vi "Get User Input.vi"(10 "OK Button Text":string, 11 "Sequence Context In":refnum<k7>) -> (1 "Continue Testing?":bool, 2 "UUT Data":T2)   [LabVIEW 2010]
uses:
  TouchScreen UI Elements/_TypeDefs/OK Button_TouchScreen.ctl
  Data to Validate.ctl
  <vilib>/addons/TestStand/_TSUtility.llb/TestStand - Get Property Value (String).vi
panel:
  in  "Work Order Number":string
  in  "QiG Serial Number":string
  in  "UUT Part Number":string
  in  "Cancel Button":T1
  in  "Continue Button":T1
  in  "UUT MICS ID":u32 format="%06x"
  in  "UUT Serial Number":string
  in  "UUT Lot Number":string
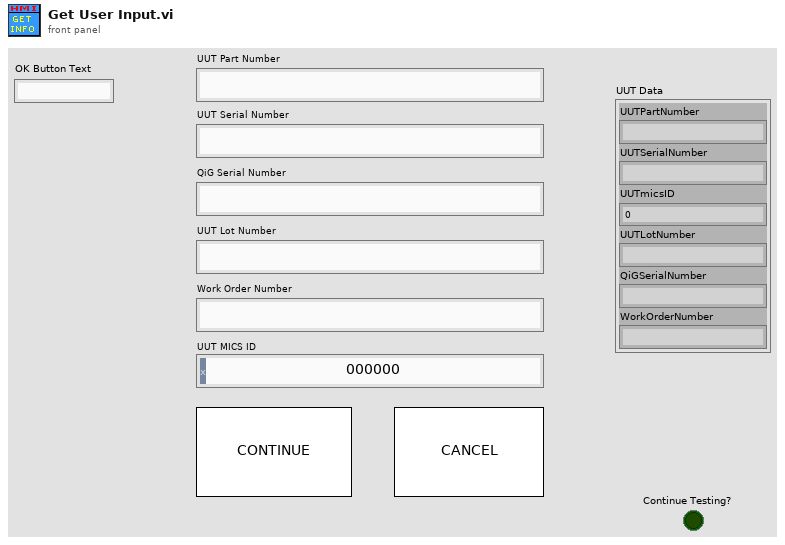
[diagram p1: front panel]
types:
  T1 = typedef "OK Button_TouchScreen.ctl" = bool
  T2 = cluster{"UUTmicsID":u32, "UUTLotNumber":string, "UUTSerialNumber":string, "UUTPartNumber":string, "QiGSerialNumber":string, "WorkOrderNumber":string}
  T3 = enum32{"Invalid", "Standard", "Closed", "Hidden", "Minimized", "Maximized"}
  T4 = typedef "Data to Validate.ctl" = enum16{"UUT_Part_Number", "UUT_Serial_Number", "QiG_Serial_Number", "UUT_Model_Number", "UUT_Lot_Number", "Work_Order_Number", "UUT_MICS_ID"}
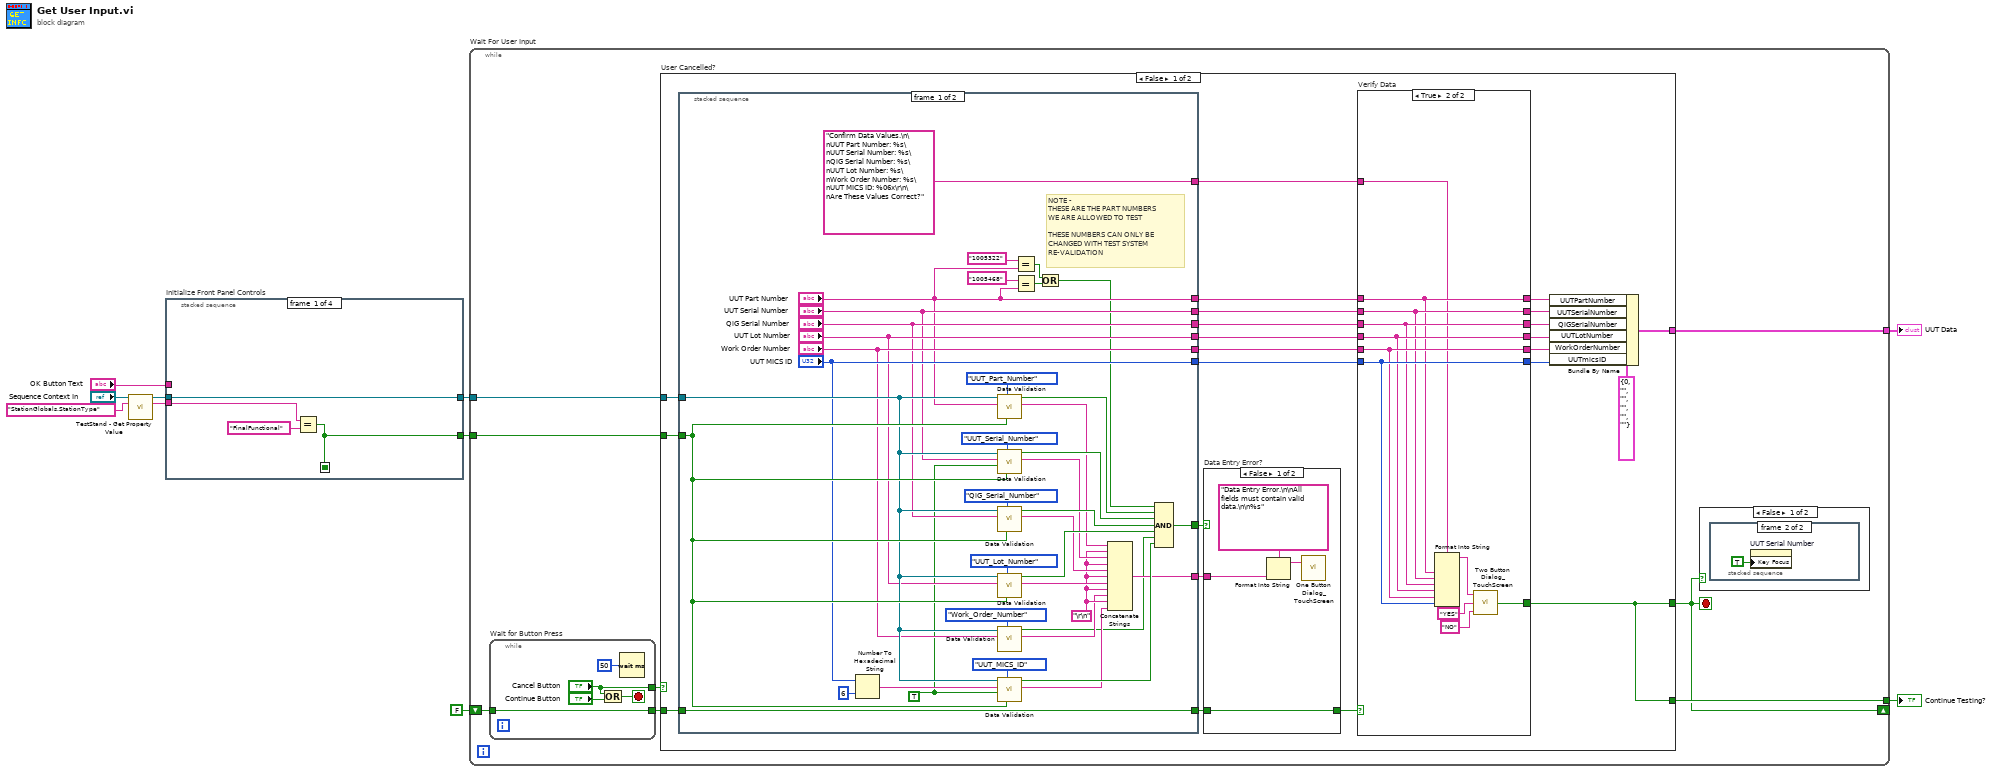
[diagram p0: block diagram]
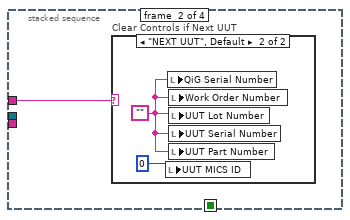
[diagram p2: hidden frame]
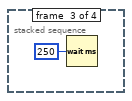
[diagram p4: hidden frame]
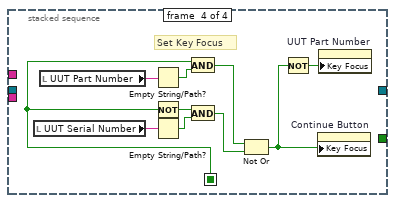
[diagram p5: hidden frame]
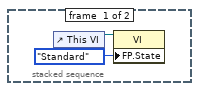
[diagram p6: hidden frame]
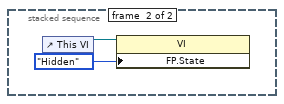
[diagram p8: hidden frame]
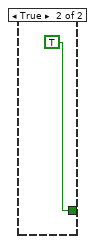
[diagram p10: hidden frame]
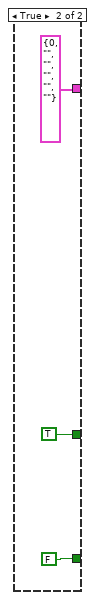
[diagram p11: hidden frame]
diagram:
  n1 = call-poly <vilib>:"TestStand - Get Property Value.vi"("Sequence Context In"="Sequence Context In", "Lookup String"="StationGlobals.StationType") -> ("Sequence Context Out"=w4:refnum<k7>, "Value"=w3:string)  [unwired: 11 in, 1 out]
  n2 = stacked-sequence "Initialize Front Panel Controls" {
    seq-local: [w11 _ _ _] -> [_ _ _ w24]
    tunnel: "OK Button Text" -> [_ w15 _ _]
    tunnel: w4 -> [w14 _ _ _]
    tunnel: w3 -> [w13 _ _ _]
    tunnel: [w14 _ _ _] -> w2
    tunnel: [w11 _ _ _] -> w1
    frame #0 {
      n3 = Equal?(x=w13, y="FinalFunctional") -> (x = y?=w11:bool)
    }
    frame #1 {
      n4 = case "Clear Controls if Next UUT" shown="\"NEXT UUT\", Default" w15 {
        frame "RETEST" {
        }
        frame "NEXT UUT", Default {
          w16 = "" ("Device LOT Number")
          n5 = local write "UUT MICS ID"(u32 0 ("Device MICS ID")) -> ()
          n6 = local write "QiG Serial Number"(w16) -> ()
          n7 = local write "Work Order Number"(w16) -> ()
          n8 = local write "UUT Lot Number"(w16) -> ()
          n9 = local write "UUT Serial Number"(w16) -> ()
          n10 = local write "UUT Part Number"(w16) -> ()
        }
      }
    }
    frame #2 {
      n11 = Wait (ms)(milliseconds to wait=u32 250) -> ()  [unwired: 1 out]
    }
    frame #3 {
      # "Set Key Focus"
      n12 = local read "UUT Serial Number"() -> (w26:string)
      n13 = local read "UUT Part Number"() -> (w27:string)
      n14 = Empty String/Path?(string/path=w27) -> (empty?=w28:bool)
      n15 = Not(x=w24) -> (.not. x?=w23:bool)
      n16 = Empty String/Path?(string/path=w26) -> (empty?=w25:bool)
      n17 = And(x=w24, y=w28) -> (x .and. y?=w21:bool)
      n18 = And(x=w23, y=w25) -> (x .and. y?=w22:bool)
      n19 = Not Or(1:w22, 2:w21) -> (0:w19:bool)
      n20 = Not(x=w19) -> (.not. x?=w20:bool)
      n21 = property on="Continue Button" class="Bool"("Key Focus"=w19) -> ()  [unwired: 2 in, 2 out]
      n22 = property on="UUT Part Number" class="Str"("Key Focus"=w20) -> ()  [unwired: 2 in, 2 out]
    }
  }
  n23 = while "Wait For User Input" {
    shift-right: [w31] -> _
    shift-left: FALSE -> [w36]
    tunnel: [w34] -> w7
    tunnel: [w32] -> w9
    tunnel: w2 -> [w30]
    tunnel: w1 -> [w29]
    stop <- w31 stop-if-true
    n24 = while "Wait for Button Press" {
      tunnel: w36 -> [w134]
      tunnel: [w134] -> w35
      tunnel: ["Cancel Button"] -> w33
      stop <- w131 stop-if-true
      n25 = Or(x="Cancel Button", y="Continue Button") -> (x .or. y?=w131:T1)
      n26 = Wait (ms)(milliseconds to wait=u32 50) -> ()  [unwired: 1 out]
    }
    n27 = case "User Cancelled?" shown="False" w33 {
      tunnel: w35 -> [w61 _]
      tunnel: [w51 TRUE ("T button?")] -> w31
      tunnel: [w56 T2 {"UUTmicsID"=0, "UUTLotNumber"="", "UUTSerialNumber"="", "UUTPartNumber"="", "QiGSerialNumber"="", "WorkOrderNumber"=""} ("UUT Data")] -> w34
      tunnel: [w51 FALSE] -> w32
      tunnel: w30 -> [w49 _]
      tunnel: w29 -> [w46 _]
      frame False {
        n28 = stacked-sequence {
          tunnel: [w100 _] -> w62
          tunnel: ["UUT Serial Number" _] -> w57
          tunnel: ["UUT Lot Number" _] -> w58
          tunnel: ["UUT MICS ID" _] -> w54
          tunnel: w61 -> [w99 _]
          tunnel: [w99 _] -> w60
          tunnel: [w87 _] -> w50
          tunnel: w49 -> [w75 _]
          tunnel: ["UUT Part Number" _] -> w48
          tunnel: w46 -> [w81 _]
          tunnel: ["Confirm Data Values.\n\nUUT Part Number: %s\nUUT Serial Number: %s\nQiG Serial Number: %s\nUUT Lot Number: %s\nWork Order Number: %s\nUUT MICS ID: %06x\r\n\nAre These Values Correct?" ("format string") _] -> w45
          tunnel: ["QiG Serial Number" _] -> w44
          tunnel: ["Work Order Number" _] -> w43
          frame #0 {
            w78 = "\r\n"
            w63 = TRUE
            # "NOTE -\nTHESE ARE THE PART NUMBERS\nWE ARE ALLOWED TO TEST\n\nTHESE NUMBERS CAN ONLY BE\nCHANGED WITH TEST SYSTEM\nRE-VALIDATION"
            n29 = Number To Hexadecimal String(1:i16 6 ("width (-)"), 2:"UUT MICS ID") -> (0:w93:string)
            n30 = call "Data Validation.vi"("Final Functional Test Station?"=w81, "Input Data Descriptor"=Data_to_Validate."UUT_Part_Number", "Input to Validate"="UUT Part Number", "Sequence Context In"=w75) -> ("Message"=w85:string, "String Valid?"=w84:bool)  [unwired: 5 in, 1 out]
            n31 = call "Data Validation.vi"("Final Functional Test Station?"=w81, "Input Data Descriptor"=Data_to_Validate."UUT_Serial_Number", "Is HEX String?"=w63, "Input to Validate"="UUT Serial Number", "Sequence Context In"=w75) -> ("Message"=w90:string, "String Valid?"=w97:bool)  [unwired: 4 in, 1 out]
            n32 = call "Data Validation.vi"("Final Functional Test Station?"=w81, "Input Data Descriptor"=Data_to_Validate."QiG_Serial_Number", "Input to Validate"="QiG Serial Number", "Sequence Context In"=w75) -> ("Message"=w79:string, "String Valid?"=w101:bool)  [unwired: 5 in, 1 out]
            n33 = call "Data Validation.vi"("Final Functional Test Station?"=w81, "Input Data Descriptor"=Data_to_Validate."UUT_Lot_Number", "Input to Validate"="UUT Lot Number", "Sequence Context In"=w75) -> ("Message"=w89:string, "String Valid?"=w95:bool)  [unwired: 5 in, 1 out]
            n34 = call "Data Validation.vi"("Input Data Descriptor"=Data_to_Validate."Work_Order_Number", "Input to Validate"="Work Order Number", "Sequence Context In"=w75) -> ("Message"=w77:string, "String Valid?"=w76:bool)  [unwired: 6 in, 1 out]
            n35 = call "Data Validation.vi"("Final Functional Test Station?"=w81, "Input Data Descriptor"=Data_to_Validate."UUT_MICS_ID", "Is HEX String?"=w63, "Input to Validate"=w93, "Sequence Context In"=w75) -> ("Message"=w88:string, "String Valid?"=w91:bool)  [unwired: 4 in, 1 out]
            n36 = Equal?(x="1005322" ("Message"), y="UUT Part Number") -> (x = y?=w65:bool)
            n37 = Equal?(x="1005468" ("Message"), y="UUT Part Number") -> (x = y?=w66:bool)
            n38 = Or(x=w65, y=w66) -> (x .or. y?=w64:bool)
            n39 = Concatenate Strings(w85, w78, w90, w78, w79, w78, w89, w78, w77, w78, w88) -> (w87:string)
            n40 = Compound Arithmetic op=AND(w64, w84, w97, w101, w95, w76, w91) -> (w100:bool)
          }
          frame #1 {
            n41 = control-ref of="This VI"() -> (w103:refnum<vi>)
            n42 = property class="VI"(reference=w103, "FP.State"=T3."Hidden" ("Front Panel Window:State")) -> ()  [unwired: 1 in, 2 out]
          }
        }
        n43 = case "Data Entry Error?" shown="False" w62 {
          tunnel: w60 -> [w125 _]
          tunnel: [w125 TRUE] -> w59
          tunnel: w50 -> [w122 _]
          frame False {
            n44 = Format Into String(format string="Data Entry Error.\n\nAll fields must contain valid data.\n\n%s" ("message"), w122) -> (resulting string=w123:string)  [unwired: 2 in, 1 out]
            n45 = call "One Button Dialog_TouchScreen.vi"("Message"=w123) -> ()  [unwired: 1 in, 1 out]
          }
          frame True {
          }
        }
        n46 = case "Verify Data" shown="True" w59 {
          selector: w59 -> [w107 _]
          tunnel: w54 -> [w110 w117]
          tunnel: w58 -> [w109 w115]
          tunnel: w57 -> [w108 w113]
          tunnel: [w107 w118] -> w51
          tunnel: [w110 w117] -> w53
          tunnel: [w109 w115] -> w55
          tunnel: [w108 w113] -> w52
          tunnel: w48 -> [w106 w112]
          tunnel: [w106 w112] -> w47
          tunnel: w45 -> [_ w111]
          tunnel: w44 -> [w105 w114]
          tunnel: w43 -> [w104 w116]
          tunnel: [w105 w114] -> w40
          tunnel: [w104 w116] -> w41
          frame False {
          }
          frame True {
            n47 = Format Into String(format string=w111, w112, w113, w114, w115, w116, w117) -> (resulting string=w121:string)  [unwired: 2 in, 1 out]
            n48 = call "Two Button Dialog_TouchScreen.vi"("F button name (\"Cancel\")"="NO" ("F button name (\"Cancel\")"), "T button name (\"OK\")"="YES" ("T button name (\"OK\")"), "Message"=w121) -> ("T Button?"=w118:T1)
          }
        }
        n49 = Bundle By Name(cluster=T2 {"UUTmicsID"=0, "UUTLotNumber"="", "UUTSerialNumber"="", "UUTPartNumber"="", "QiGSerialNumber"="", "WorkOrderNumber"=""} ("UUT Data"), "UUTPartNumber"=w47, "UUTSerialNumber"=w52, "QiGSerialNumber"=w40, "UUTLotNumber"=w55, "WorkOrderNumber"=w41, "UUTmicsID"=w53) -> (w56:T2)
      }
      frame True {
      }
    }
    n50 = case shown="False" w31 {
      frame False {
        n51 = stacked-sequence {
          frame #0 {
            n52 = control-ref of="This VI"() -> (w38:refnum<vi>)
            n53 = property class="VI"(reference=w38, "FP.State"=T3."Standard" ("Front Panel Window:State")) -> ()  [unwired: 1 in, 2 out]
          }
          frame #1 {
            n54 = property on="UUT Serial Number" class="Str"("Key Focus"=TRUE) -> ()  [unwired: 2 in, 2 out]
          }
        }
      }
      frame True {
      }
    }
  }
  "UUT Data" <- w7
  "Continue Testing?" <- w9
